vi "SetTemp_popup.vi"(0 "Input Line Command":string, 1 "Device List":string(combo)="LS336", 3 "error in (no error)":errorcluster, 4 "Output":string(combo)="1", 5 "Temperature (K)":string, 6 "VISA":refnum<visa-resource-name>, 7 "Rate (K/min)":string="0") -> (8 "error out":errorcluster, 9 "Cancel":bool, 10 "Output Line Command":string)   [LabVIEW 2020]
panel:
  in  "platform":u16(ring) items=["Mac", "PC"]
  in  "Cancel Button":bool
  in  "OK Button":bool
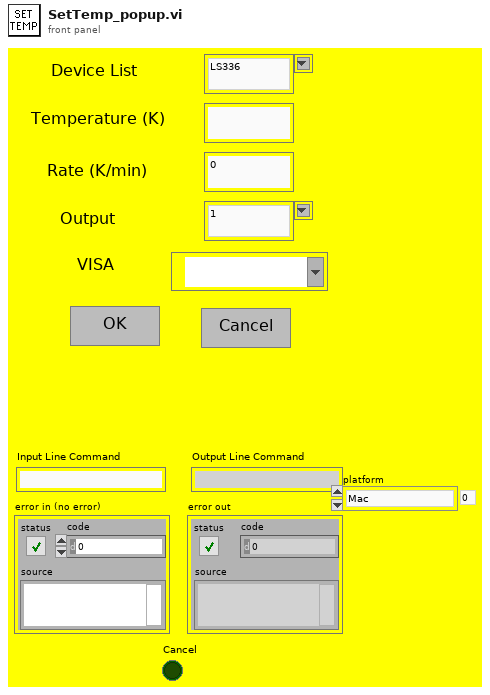
[diagram p1: front panel]
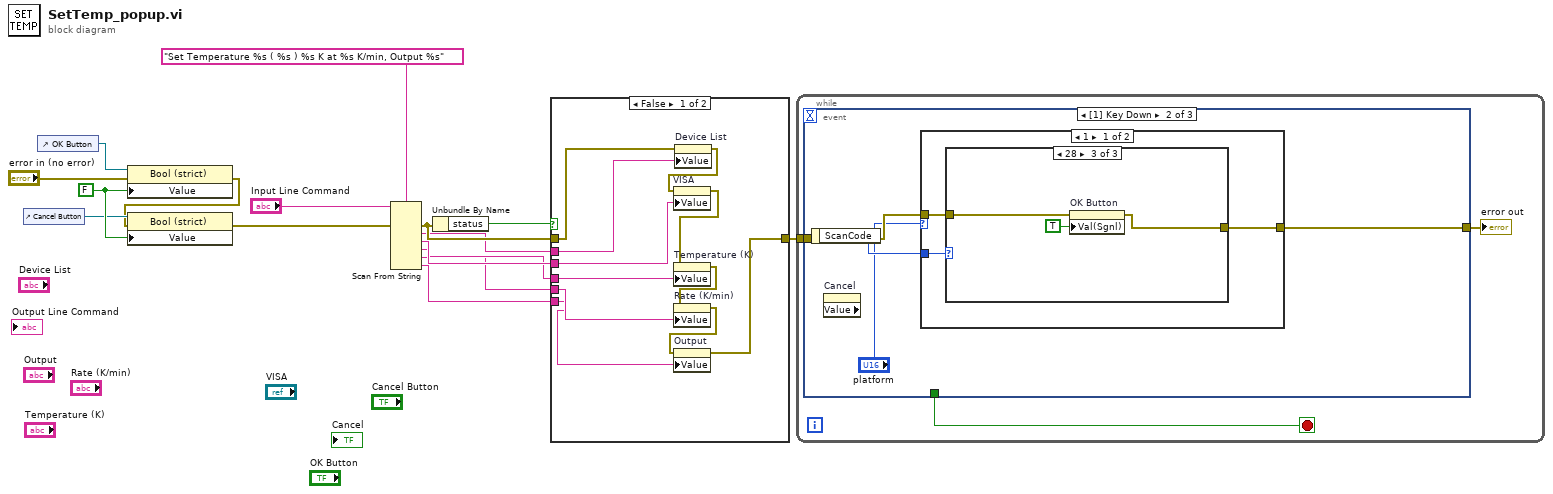
[diagram p0: block diagram]
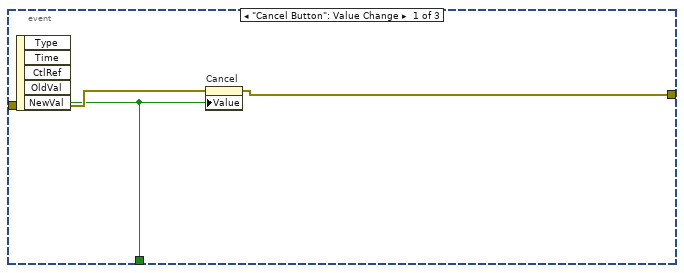
[diagram p2: hidden frame]
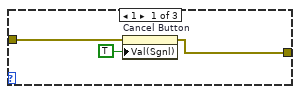
[diagram p3: hidden frame]
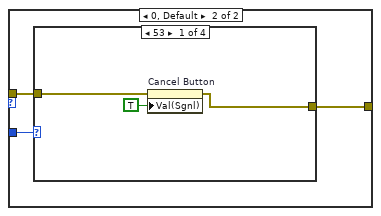
[diagram p5: hidden frame]
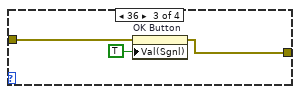
[diagram p7: hidden frame]
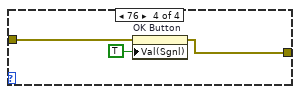
[diagram p8: hidden frame]
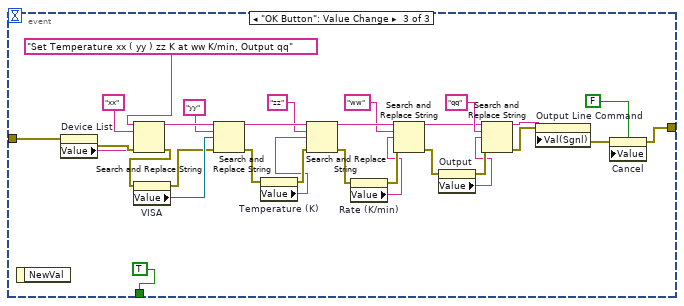
[diagram p9: hidden frame]
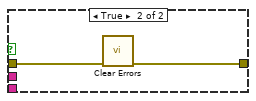
[diagram p10: hidden frame]
diagram:
  w14 = FALSE
  n1 = control-ref of="Cancel Button"() -> (w13:refnum<vi>)
  n2 = control-ref of="OK Button"() -> (w15:refnum<vi>)
  n3 = property on="Property Node" class="Bool (strict)"(reference=w15, error in="error in (no error)", "Value"=w14) -> (error out=w12:errorcluster)  [unwired: 1 out]
  n4 = property on="Property Node" class="Bool (strict)"(reference=w13, error in=w12, "Value"=w14) -> (error out=w11:errorcluster)  [unwired: 1 out]
  n5 = Scan From String(format string="Set Temperature %s ( %s ) %s K at %s K/min, Output %s", input string="Input Line Command", error in=w11) -> (error out=w7:errorcluster, output 1=w6:string, output 2=w5:string, output 3=w4:string, output 4=w3:string, output 5=w2:string)  [unwired: 6 in, 2 out]
  n6 = Unbundle By Name(w7) -> ("status"=w8:bool)
  n7 = case shown="False" w8 {
    tunnel: w7 -> [w27 w29]
    tunnel: [w17 w28] -> w1
    tunnel: w6 -> [w26 _]
    tunnel: w5 -> [w24 _]
    tunnel: w4 -> [w22 _]
    tunnel: w3 -> [w20 _]
    tunnel: w2 -> [w19 _]
    frame False {
      n8 = property on="Device List" class="CmbBox"(error in=w27, "Value"=w26) -> (error out=w25:errorcluster)  [unwired: 1 in, 1 out]
      n9 = property on="VISA" class="VISAName"(error in=w25, "Value"=w24) -> (error out=w23:errorcluster)  [unwired: 1 in, 1 out]
      n10 = property on="Temperature (K)" class="Str"(error in=w23, "Value"=w22) -> (error out=w21:errorcluster)  [unwired: 1 in, 1 out]
      n11 = property on="Rate (K/min)" class="Str"(error in=w21, "Value"=w20) -> (error out=w18:errorcluster)  [unwired: 1 in, 1 out]
      n12 = property on="Output" class="CmbBox"(error in=w18, "Value"=w19) -> (error out=w17:errorcluster)  [unwired: 1 in, 1 out]
    }
    frame True {
      n13 = call <vilib>:"Clear Errors.vi"("error in (no error)"=w29) -> ("error out"=w28:errorcluster)  [unwired: 5 in, 1 out]
    }
  }
  n14 = while {
    tunnel: w1 -> [w32]
    stop <- w31 stop-if-true
    n15 = event shown="[1] Key Down" {
      selector: _ -> [_ _ _]
      dyn-events: _ -> [_ _ _]
      timeout: _ -> [_ _ _]
      tunnel: w32 -> [w35 w38 w91]
      tunnel: [w34 _ TRUE] -> w31
      tunnel: [w33 w37 w64] -> w30
      event "Cancel Button": Value Change {
        n16 = event-data() -> ("NewVal"=w34:bool)  [unwired: 1 in, 4 out]
        n17 = property on="Cancel" class="Bool (strict)"(error in=w35, "Value"=w34) -> (error out=w33:errorcluster)  [unwired: 1 in, 1 out]
      }
      event Key Down {
        n18 = event-data() -> ("ScanCode"=w39:i16)  [unwired: 1 in]
        n19 = property on="Cancel" class="Bool (strict)" props=["Value"]() -> ()  [unwired: 2 in, 3 out]
        n20 = case shown="1" "platform" {
          tunnel: w39 -> [w42 w52]
          tunnel: w38 -> [w41 w51]
          tunnel: [w40 w50] -> w37
          frame 1 {
            n21 = case shown="28" w42 {
              tunnel: w41 -> [w45 w46 w48]
              tunnel: [w43 w46 w47] -> w40
              frame 1 {
                n22 = property on="Cancel Button" class="Bool (strict)"(error in=w45, "Val(Sgnl)"=TRUE ("Value (Signaling)")) -> (error out=w43:errorcluster)  [unwired: 1 in, 1 out]
              }
              frame Default {
              }
              frame 28 {
                n23 = property on="OK Button" class="Bool (strict)"(error in=w48, "Val(Sgnl)"=TRUE ("Value (Signaling)")) -> (error out=w47:errorcluster)  [unwired: 1 in, 1 out]
              }
            }
          }
          frame 0, Default {
            n24 = case shown="53" w52 {
              tunnel: w51 -> [w55 w56 w58 w61]
              tunnel: [w53 w56 w57 w60] -> w50
              frame 53 {
                n25 = property on="Cancel Button" class="Bool (strict)"(error in=w55, "Val(Sgnl)"=TRUE ("Value (Signaling)")) -> (error out=w53:errorcluster)  [unwired: 1 in, 1 out]
              }
              frame Default {
              }
              frame 36 {
                n26 = property on="OK Button" class="Bool (strict)"(error in=w58, "Val(Sgnl)"=TRUE ("Value (Signaling)")) -> (error out=w57:errorcluster)  [unwired: 1 in, 1 out]
              }
              frame 76 {
                n27 = property on="OK Button" class="Bool (strict)"(error in=w61, "Val(Sgnl)"=TRUE ("Value (Signaling)")) -> (error out=w60:errorcluster)  [unwired: 1 in, 1 out]
              }
            }
          }
        }
      }
      event "OK Button": Value Change {
        n28 = event-data() -> ()  [unwired: 1 in, 1 out]
        n29 = property on="Device List" class="CmbBox"(error in=w91) -> (error out=w90:errorcluster, "Value"=w89:string)  [unwired: 1 in, 1 out]
        n30 = Search and Replace String(input string="Set Temperature xx ( yy ) zz K at ww K/min, Output qq" ("format string"), search string="xx", replace string=w89, error in=w90) -> (result string=w88:string, error out=w83:errorcluster)  [unwired: 4 in, 2 out]
        n31 = property on="VISA" class="VISAName"(error in=w83) -> (error out=w82:errorcluster, "Value"=w86:refnum<visa-resource-name>)  [unwired: 1 in, 1 out]
        n32 = Search and Replace String(input string=w88, search string="yy", replace string=w86, error in=w82) -> (result string=w85:string, error out=w81:errorcluster)  [unwired: 4 in, 2 out]
        n33 = property on="Temperature (K)" class="Str"(error in=w81) -> (error out=w80:errorcluster, "Value"=w79:string)  [unwired: 1 in, 1 out]
        n34 = Search and Replace String(input string=w85, search string="zz", replace string=w79, error in=w80) -> (result string=w78:string, error out=w76:errorcluster)  [unwired: 4 in, 2 out]
        n35 = property on="Rate (K/min)" class="Str"(error in=w76) -> (error out=w75:errorcluster, "Value"=w74:string)  [unwired: 1 in, 1 out]
        n36 = Search and Replace String(input string=w78, search string="ww", replace string=w74, error in=w75) -> (result string=w72:string, error out=w71:errorcluster)  [unwired: 4 in, 2 out]
        n37 = property on="Output" class="CmbBox"(error in=w71) -> (error out=w70:errorcluster, "Value"=w69:string)  [unwired: 1 in, 1 out]
        n38 = Search and Replace String(input string=w72, search string="qq", replace string=w69, error in=w70) -> (result string=w67:string, error out=w68:errorcluster)  [unwired: 4 in, 2 out]
        n39 = property on="Output Line Command" class="Str"(error in=w68, "Val(Sgnl)"=w67) -> (error out=w65:errorcluster)  [unwired: 1 in, 1 out]
        n40 = property on="Cancel" class="Bool (strict)"(error in=w65, "Value"=FALSE ("Cancel")) -> (error out=w64:errorcluster)  [unwired: 1 in, 1 out]
      }
    }
    "error out" <- w30
  }
